vi "TelemetryServer_MultiplexerPump.vi"(3 "Multiplexer in":T1, 9 "Error out":errorcluster caption="error in (no error)") -> (0 "Multiplexer out":T1, 2 "Waveforms":waveform(dbl)[](array[waveform]), 6 "error in":errorcluster caption="error out")   [LabVIEW 2009]
uses:
  <vilib>/Waveform/WDTOps.llb/WDT Get Final Time Value DBL.vi
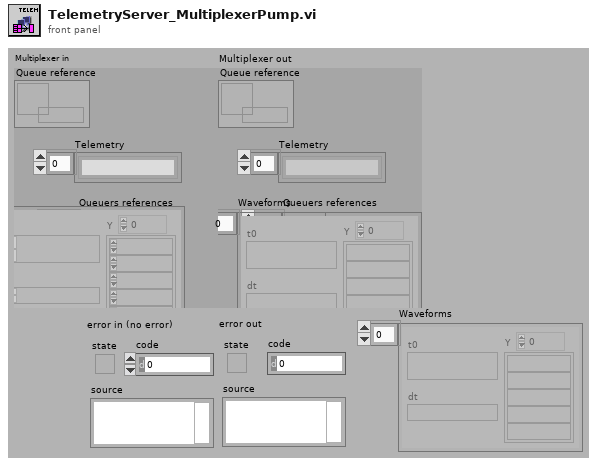
[diagram p1: front panel]
types:
  T1 = cluster{"Queue reference":refnum<queue>, "Telemetry":string[], "Queuers references":refnum<vi>[], "Waveforms":waveform(dbl)[]}
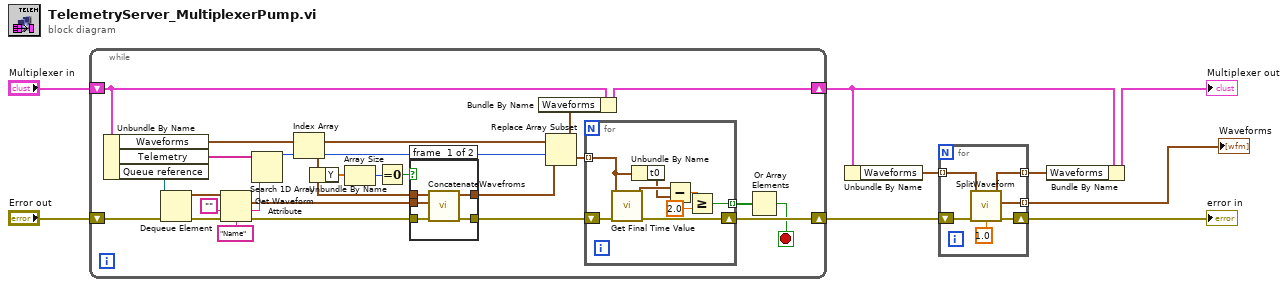
[diagram p0: block diagram]
diagram:
  n1 = while {
    shift-right: [w23] -> w7
    shift-left: "Error out" -> [w33]
    shift-right: [w20] -> w3
    shift-left: "Multiplexer in" -> [w21]
    stop <- w18 stop-if-true
    n2 = Unbundle By Name(w21) -> ("Waveforms"=w25:waveform(dbl)[], "Telemetry"=w27:string[], "Queue reference"=w30:refnum<queue>)
    n3 = Dequeue Element(queue=w30, error in (no error)=w33) -> (element=w28:waveform(dbl), error out=w29:errorcluster)  [unwired: 3 out]
    n4 = Get Waveform Attribute(4:w29, 5:"", 6:"Name" ("nom"), 7:w28) -> (0:w14:errorcluster, 1:w26:string, 3:w17:waveform(dbl))  [unwired: 1 out]
    n5 = Search 1D Array(1D array=w27, element=w26) -> (index of element=w24:i32)  [unwired: 1 out]
    n6 = Index Array(array=w25, index=w24) -> (element=w13:waveform(dbl))
    n7 = Unbundle By Name(w13) -> ("Y"=w16:dbl[])
    n8 = Array Size(array=w16) -> (size(s)=w15:i32)
    n9 = Equal To 0?(x=w15) -> (x = 0?=w12:bool)
    n10 = case shown="False" w12 {
      tunnel: w17 -> [w34 w40]
      tunnel: w14 -> [w38 w39]
      tunnel: w13 -> [w35 _]
      tunnel: [w36 w40] -> w10
      tunnel: [w37 w39] -> w11
      frame #0 {
        n11 = call "ConcatenateWavefroms.vi"("waveform A"=w35, "waveform B"=w34, "error in (no error)"=w38) -> ("Graphe"=w36:waveform(dbl), "error out"=w37:errorcluster)  [unwired: 5 out]
      }
      frame #1 {
      }
    }
    n12 = Replace Array Subset(array=w25, new element=w10, index=w24) -> (w22:waveform(dbl)[])
    n13 = Bundle By Name(cluster=w21, "Waveforms"=w22) -> (w20:T1)
    n14 = for {
      shift-right: [w47] -> w23
      shift-left: w11 -> [w48]
      tunnel: w22 -> [w42] mode=indexing
      tunnel: [w44] -> w19 mode=indexing
      n15 = call-poly <vilib>:"Get Final Time Value.vi"("error in (no error)"=w48, "waveform in"=w42) -> ("error out"=w47:errorcluster, "tf"=w43:timestamp)  [unwired: 8 out]
      n16 = Unbundle By Name(w42) -> ("t0"=w41:timestamp)
      n17 = Subtract(x=w43, y=w41) -> (x-y=w46:dbl)
      n18 = Greater Or Equal?(x=w46, y=2.0) -> (x >= y?=w44:bool)
    }
    n19 = Or Array Elements(Boolean array=w19) -> (logical OR=w18:bool)
  }
  n20 = Unbundle By Name(w3) -> ("Waveforms"=w6:waveform(dbl)[])
  n21 = for {
    shift-right: [w53] -> w4
    shift-left: w7 -> [w54]
    tunnel: w6 -> [w49] mode=indexing
    tunnel: [w51] -> w5 mode=indexing
    tunnel: [w50] -> w1 mode=indexing
    n22 = call "SplitWaveform.vi"("signal in"=w49, "Duration"=1.0, "error in (no error)"=w54) -> ("last signal out"=w50:waveform(dbl), "first signal out"=w51:waveform(dbl), "error out"=w53:errorcluster)  [unwired: 4 out]
  }
  "error in" <- w4
  "Waveforms" <- w5
  n23 = Bundle By Name(cluster=w3, "Waveforms"=w1) -> (→"Multiplexer out":T1)
